vi "TimedMessageToUser.vi"(7 "condition":enum16{"Notify", "Status", "Error", "Warning"}(ring), 10 "Notify":string) -> ()   [LabVIEW 2011]
panel:
  in  "OK Button 2":bool
  in  "OK Button":bool
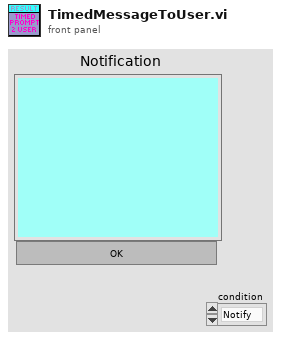
[diagram p1: front panel]
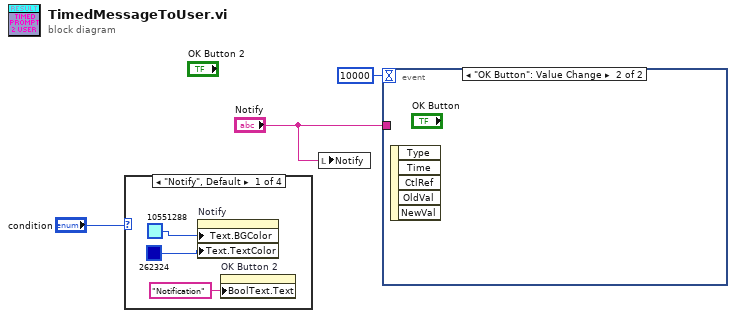
[diagram p0: block diagram]
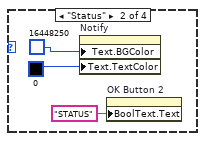
[diagram p2: hidden frame]
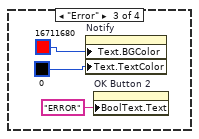
[diagram p3: hidden frame]
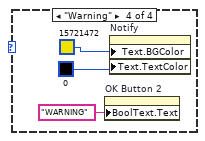
[diagram p4: hidden frame]
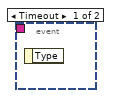
[diagram p5: hidden frame]
diagram:
  n1 = case shown="\"Notify\", Default" "condition" {
    frame "Notify", Default {
      n2 = property on="Notify" class="Str"("Text.BGColor"=u32 10551288 ("Color Box"), "Text.TextColor"=u32 262324 ("Color Box")) -> ()  [unwired: 2 in, 2 out]
      n3 = property on="OK Button 2" class="Bool"("BoolText.Text"="Notification" ("Boolean Text.Text")) -> ()  [unwired: 2 in, 2 out]
    }
    frame "Status" {
      n4 = property on="Notify" class="Str"("Text.BGColor"=u32 16448250 ("Color Box"), "Text.TextColor"=u32 0 ("Color Box")) -> ()  [unwired: 2 in, 2 out]
      n5 = property on="OK Button 2" class="Bool"("BoolText.Text"="STATUS" ("Boolean Text.Text")) -> ()  [unwired: 2 in, 2 out]
    }
    frame "Error" {
      n6 = property on="Notify" class="Str"("Text.BGColor"=u32 16711680 ("Color Box"), "Text.TextColor"=u32 0 ("Color Box")) -> ()  [unwired: 2 in, 2 out]
      n7 = property on="OK Button 2" class="Bool"("BoolText.Text"="ERROR" ("Boolean Text.Text")) -> ()  [unwired: 2 in, 2 out]
    }
    frame "Warning" {
      n8 = property on="OK Button 2" class="Bool"("BoolText.Text"="WARNING" ("Boolean Text.Text")) -> ()  [unwired: 2 in, 2 out]
      n9 = property on="Notify" class="Str"("Text.BGColor"=u32 15721472 ("Color Box"), "Text.TextColor"=u32 0 ("Color Box")) -> ()  [unwired: 2 in, 2 out]
    }
  }
  n10 = local write "Notify"("Notify") -> ()
  n11 = event shown="[1] \"OK Button\": Value Change" {
    selector: _ -> [_ _]
    dyn-events: _ -> [_ _]
    timeout: 10000 -> [_ _]
    tunnel: "Notify" -> [_ _]
    event Timeout {
      n12 = event-data() -> ()  [unwired: 1 in, 1 out]
    }
    event "OK Button": Value Change {
      n13 = event-data() -> ()  [unwired: 1 in, 5 out]
    }
  }
